vi "Split name and data.vi"(11 "string":string) -> (2 "Data":string, 3 "Command Name":string)   [LabVIEW 2013]
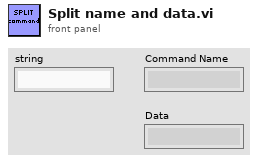
[diagram p1: front panel]
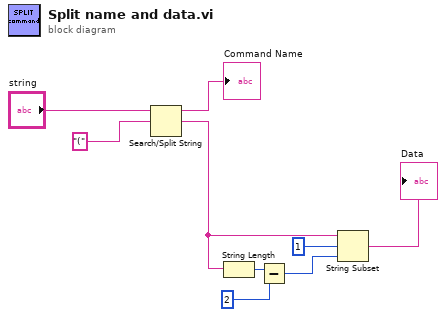
[diagram p0: block diagram]
diagram:
  n1 = Search/Split String(string="string", search string/char (-)="(") -> (substring before match=→"Command Name":string, match + rest of string=w4:string)  [unwired: 1 in, 1 out]
  n2 = String Length(string=w4) -> (length=w3:i32)
  n3 = Subtract(x=w3, y=2) -> (x-y=w2:i32)
  n4 = String Subset(string=w4, offset (0)=1, length (rest)=w2) -> (substring=→"Data":string)
